vi "XIPIN_Motion_Adaptive_Noise_Reduction_1_1.vi"   [LabVIEW 2017]
doc: "The Xilinx Motion Adaptive Noise Reduction LogiCORE is an effective module for both motion detection and motion adaptive noise reduction in video streams. The core allows the motion detection function to be used independently of the noise reduction function for applications where noise reduction is not needed. The noise reduction algorithm is implemented as a recursive temporal filter with a user programmable transfer function allowing the user to control both the shape of the motion transfer and the strength of the noise reduction applied. The motion transfer function is initialized according to the settings in the Coregen GUI, but is also programmable at runtime via the register interface. The LogiCORE is provided with two different interfaces: General purpose processor and EDK Pcore (including device driver).\n------------------------------------\n<b>Need License</b> : Yes"
uses:
  <vilib>/rvi/XilinxIP/XIPIN_XNode/niFpgaXIPIN.xnode
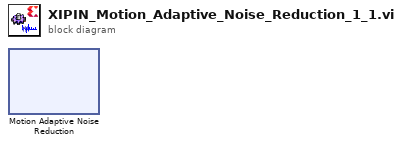
[diagram p0: block diagram]
diagram:
  n1 = xnode ("Motion Adaptive Noise Reduction")() -> ()
